vi "Chroma_PowerSupply_IDN.vi"(8 "错误输入（无错误）":errorcluster, 11 "VISA资源名称":refnum<visa-resource-name>="COM1") -> (0 "错误输出":errorcluster, 1 "读取缓冲区":string, 2 "status":bool, 3 "VISA资源名称输出":refnum<visa-resource-name>, 5 "返回数":u32)   [LabVIEW 2012]
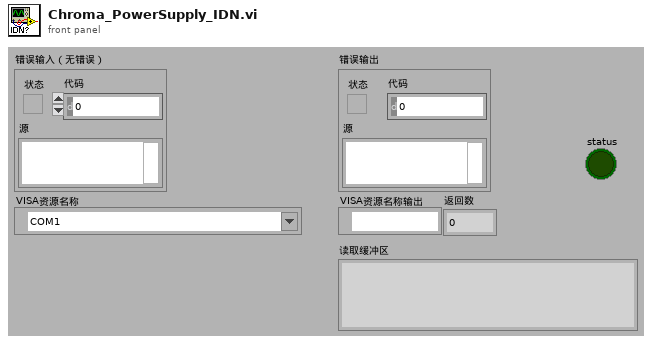
[diagram p1: front panel]
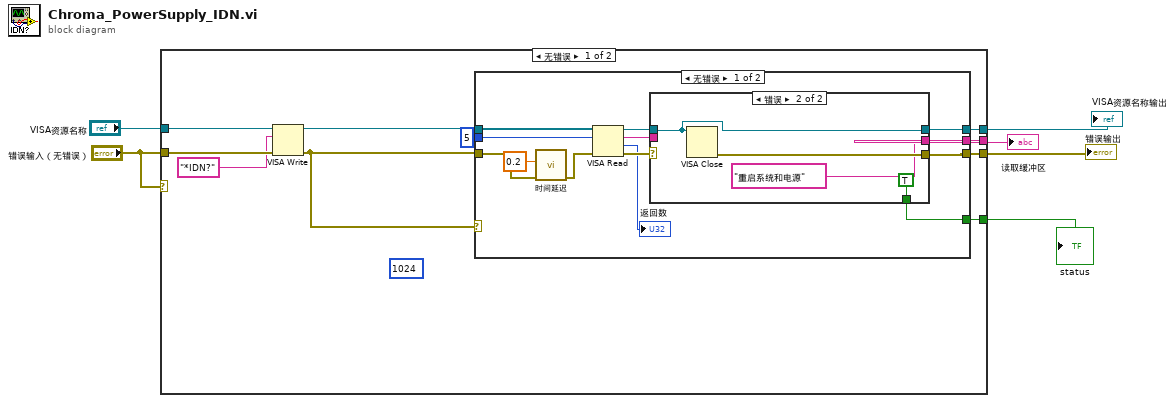
[diagram p0: block diagram]
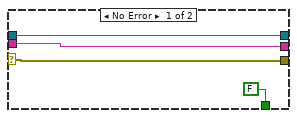
[diagram p2: hidden frame]
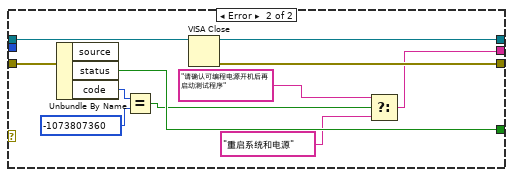
[diagram p3: hidden frame]
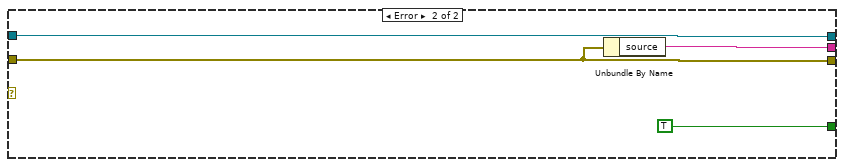
[diagram p4: hidden frame]
diagram:
  n1 = case shown="无错误" "错误输入（无错误）" {
    tunnel: [w16 w50] -> w6
    tunnel: [w15 w51] -> w5
    tunnel: [w14 w49] -> w4
    tunnel: "VISA资源名称" -> [w8 w51]
    tunnel: "错误输入（无错误）" -> [w9 w50]
    tunnel: [w11 TRUE ("status")] -> w1
    frame No Error {
      (unwired) u32 1024 ("Bytes at Port")
      n2 = VISA Write(VISA resource name=w8, write buffer="*IDN?", error in (no error)=w9) -> (VISA resource name out=w13:refnum<visa-resource-name>, error out=w10:errorcluster)  [unwired: 1 out]
      n3 = case shown="无错误" w10 {
        tunnel: [w19 w47] -> w16
        tunnel: [w23 w46] -> w15
        tunnel: [w21 w40] -> w14
        tunnel: w13 -> [w29 w46]
        tunnel: w10 -> [w27 w45]
        tunnel: u32 5 ("Bytes at Port") -> [w28 _]
        tunnel: [w24 w44] -> w11
        frame No Error {
          n4 = call "时间延迟"("error in (no error)"=w27, "Delay Time (s)"=0.2) -> ("error out"=w26:errorcluster)  [unwired: 9 out]
          n5 = VISA Read(VISA resource name=w29, byte count=w28, error in (no error)=w26) -> (VISA resource name out=w22:refnum<visa-resource-name>, read buffer=w20:string, return count=→"返回数":u32, error out=w25:errorcluster)
          n6 = case shown="错误" w25 {
            selector: w25 -> [w30 _]
            tunnel: [FALSE TRUE] -> w24
            tunnel: [w32 w35] -> w23
            tunnel: w22 -> [w32 w35]
            tunnel: [w31 "重启系统和电源"] -> w21
            tunnel: w20 -> [w31 _]
            tunnel: [w30 w37] -> w19
            frame No Error {
            }
            frame Error {
              n7 = VISA Close(VISA resource name=w35) -> (error out=w37:errorcluster)  [unwired: 1 in]
            }
          }
        }
        frame Error {
          n8 = Unbundle By Name(w45) -> ("status"=w44:bool, "code"=w42:i32)  [unwired: 1 out]
          n9 = Equal?(x=w42, y=-1073807360 ("Bytes at Port")) -> (x = y?=w39:bool)
          n10 = VISA Close(VISA resource name=w46) -> (error out=w47:errorcluster)  [unwired: 1 in]
          n11 = Select(t="请确认可编程电源开机后再启动测试程序", s=w39, f="重启系统和电源") -> (s? t:f=w40:string)
        }
      }
    }
    frame Error {
      n12 = Unbundle By Name(w50) -> ("source"=w49:string)
    }
  }
  "错误输出" <- w6
  "VISA资源名称输出" <- w5
  "读取缓冲区" <- w4
  "status" <- w1
